vi "LED card.vi"(8 "error in (no error)":errorcluster, 11 "Node Ptr":T5 format="%.0x") -> (0 "error out":errorcluster)   [LabVIEW 2014, in "SLSC configuration System Explorer.lvlib"]
uses:
  SLSC configuration System Explorer.lvlib
  <vilib>/NI Veristand/Custom Device API/Custom Device Item Ref.ctl
  Type Defs/Card Position.ctl
  Shared/SPI Utility/Slot #.ctl
  Shared/LED Backplane/Bank LED States.ctl
  Shared/LED Backplane/LED State.ctl
  Shared/Constants.vi
  <vilib>/NI Veristand/Custom Device API/Get Item Property (U16).vi
  <vilib>/NI Veristand/Custom Device API/Custom Device API.lvlib
  Shared/SLSC configuration Shared.lvlib
panel:
  in  "Bank LED States":T1
  in  "Header 2":cluster{"Section Name":string}={"Section Name"="Bank 0 Settings"}
  in  "Card Position":T3 {"Slot #" max=15}
  in  "Header":cluster{"Section Name":string}={"Section Name"="LED Backplane Settings"}
  in  "Description":string
  in  "Name":string
  # "LED 1"
  # "LED 2"
  # "LED 3"
  # "LED 4"
  # "LED 5"
  # "LED 6"
  # "LED 7"
  # "LED 8"
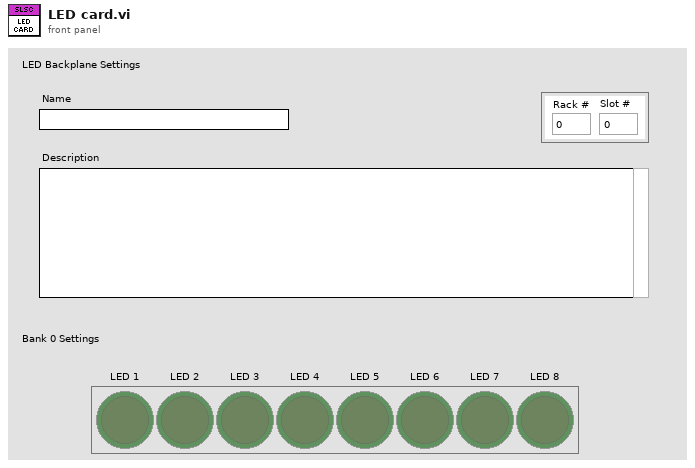
[diagram p1: front panel]
types:
  T1 = typedef "SLSC configuration Shared.lvlib/Bank LED States.ctl" = T2[]
  T2 = typedef "SLSC configuration Shared.lvlib/LED State.ctl" = bool
  T3 = typedef "SLSC configuration Shared.lvlib/Card Position.ctl" = cluster{"Rack #":u8, "Slot #":T4}
  T4 = typedef "SLSC configuration Shared.lvlib/Slot #.ctl" = u8
  T5 = typedef "Custom Device API.lvlib/Custom Device Item Ref.ctl" = u64
  T6 = typedef "Custom Device API.lvlib/Custom Device Commands.ctl" = enum16{"Default", "Item renamed", "Shutdown", "Dynamic button pressed"}
  T7 = typedef "Custom Device API.lvlib/Custom Device Item Info.ctl" = cluster{"Name":string, "Is Channel":bool, "GUID":string, "Is Waveform":bool}
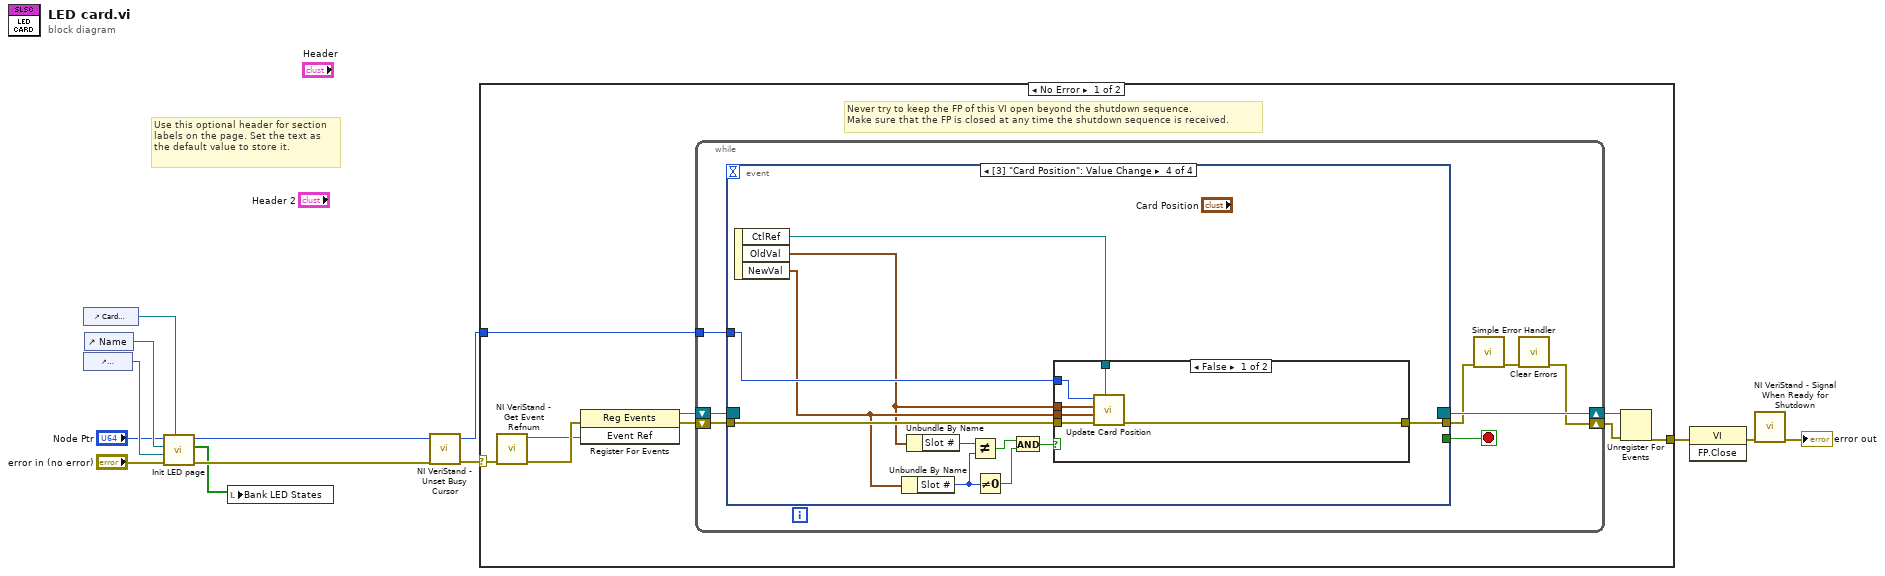
[diagram p0: block diagram]
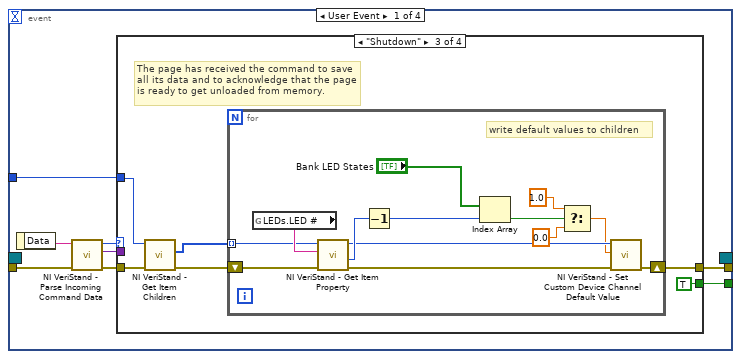
[diagram p2: hidden frame]
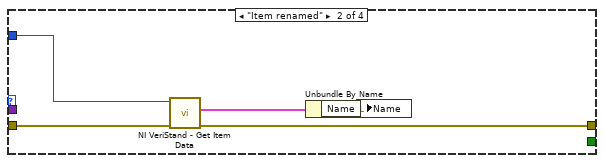
[diagram p4: hidden frame]
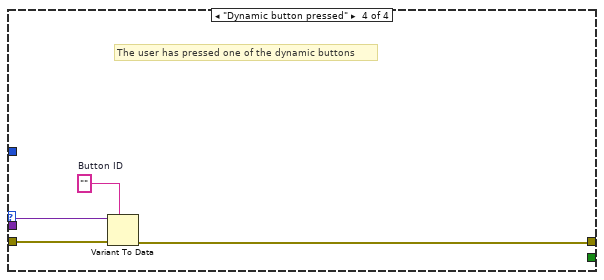
[diagram p5: hidden frame]
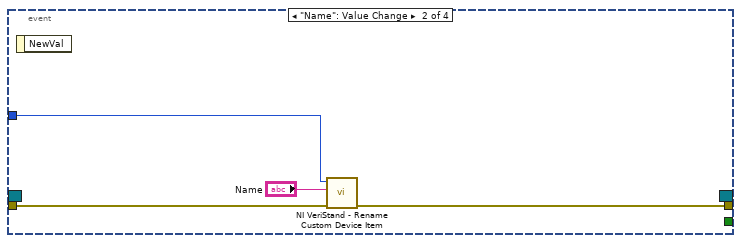
[diagram p6: hidden frame]
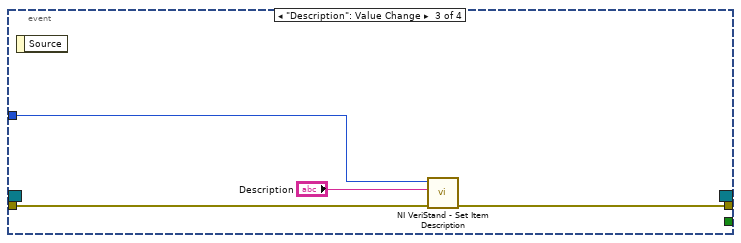
[diagram p7: hidden frame]
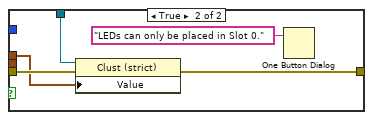
[diagram p8: hidden frame]
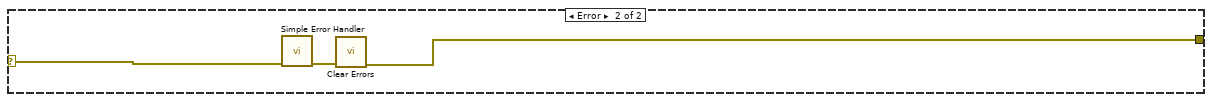
[diagram p9: hidden frame]
diagram:
  # "Use this optional header for section labels on the page. Set the text as the default value to store it."
  n1 = control-ref of="Card Position"() -> (w2:refnum<vi>)
  n2 = control-ref of="Description"() -> (w4:refnum<vi>)
  n3 = control-ref of="Name"() -> (w5:refnum<vi>)
  n4 = call "Init LED page.vi"("Card Position"=w2, "error in (no error)"="error in (no error)", "Description"=w4, "Name"=w5, "Node Ptr"="Node Ptr") -> ("error out"=w9:errorcluster, "LED States"=w1:T2[], "Node Ptr out"=w6:T5)  [unwired: 4 in]
  n5 = local write "Bank LED States"(w1) -> ()
  n6 = call <vilib>:"NI VeriStand - Unset Busy Cursor.vi"("error in (no error)"=w9) -> ("error out"=w8:errorcluster)  [unwired: 10 out]
  n7 = case shown="No Error" w8 {
    selector: w8 -> [w13 w99]
    tunnel: [w18 w97] -> w12
    tunnel: w6 -> [w14 _]
    frame No Error {
      # "Never try to keep the FP of this VI open beyond the shutdown sequence.\nMake sure that the FP is closed at any time the shutdown sequence is received."
      n8 = call <vilib>:"NI VeriStand - Get Event Refnum.vi"("error in (no error)"=w13) -> ("error out"=w21:errorcluster, "Event Ref"=w17:refnum<user-event>)  [unwired: 9 out]
      n9 = register-events(error in=w21, w17) -> (reference out=w15:refnum<event-registration>, error out=w16:errorcluster)  [unwired: 1 in]
      n10 = while {
        tunnel: w14 -> [w25]
        shift-right: [w22] -> w19
        shift-left: w16 -> [w28]
        shift-right: [w29] -> w20
        shift-left: w15 -> [w27]
        stop <- w26 stop-if-true
        n11 = event shown="[3] \"Card Position\": Value Change" {
          selector: w27 -> [_ _ _ _]
          dyn-events: [_ _ _ _] -> w29
          timeout: _ -> [_ _ _ _]
          tunnel: w28 -> [w37 w70 w73 w84]
          tunnel: [w33 _ _ _] -> w26
          tunnel: [w32 w69 w72 w85] -> w24
          tunnel: w25 -> [w31 w68 w74 w83]
          event User Event {
            n12 = event-data() -> ("Data"=w36:string)  [unwired: 1 out]
            n13 = call <vilib>:"NI VeriStand - Parse Incoming Command Data.vi"("error in (no error)"=w37, "Incoming data"=w36) -> ("error out"=w35:errorcluster, "Outgoing data"=w30:variant, "Action"=w34:T6)  [unwired: 7 out]
            n14 = case shown="\"Shutdown\"" w34 {
              tunnel: w35 -> [w38 w43 w46 w66]
              tunnel: [_ _ TRUE _] -> w33
              tunnel: [w38 w40 w48 w63] -> w32
              tunnel: w31 -> [_ w42 w44 _]
              tunnel: w30 -> [_ _ _ w65]
              frame "Default", Default {
              }
              frame "Item renamed" {
                n15 = call <vilib>:"NI VeriStand - Get Item Data.vi"("error in (no error)"=w43, "Item Ref in"=w42) -> ("error out"=w40:errorcluster, "Item Info"=w41:T7)  [unwired: 8 out]
                n16 = Unbundle By Name(w41) -> ("Name"=w39:string)
                n17 = local write "Name"(w39) -> ()
              }
              frame "Shutdown" {
                # "The page has received the command to save all its data and to acknowledge that the page is ready to get unloaded from memory."
                n18 = call <vilib>:"NI VeriStand - Get Item Children.vi"("error in (no error)"=w46, "Item Ref in"=w44) -> ("error out"=w45:errorcluster, "Child Refs"=w47:T5[])  [unwired: 6 in, 2 out]
                n19 = for {
                  shift-right: [w59] -> w48
                  shift-left: w45 -> [w61]
                  tunnel: w47 -> [w57] mode=indexing
                  # "write default values to children"
                  n20 = global read "Constants.vi" "LEDs.LED #"() -> (w62:string)
                  n21 = call-poly <vilib>:"NI VeriStand - Get Item Property.vi"("error in (no error)"=w61, "Property Name"=w62, "Item Ref in"=w57) -> ("error out"=w55:errorcluster, "Value"=w60:u16, "Item Ref out"=w58:T5)  [unwired: 5 in, 1 out]
                  n22 = Decrement(x=w60) -> (x-1=w56:u16)
                  n23 = Index Array(array="Bank LED States", index=w56) -> (element=w53:T2)
                  n24 = Select(t=1.0 ("double precision float"), s=w53, f=0.0 ("double precision float")) -> (s? t:f=w50:dbl)
                  n25 = call <vilib>:"NI VeriStand - Set Custom Device Channel Default Value.vi"("error in (no error)"=w55, "Default Value"=w50, "Channel Ref in"=w58) -> ("error out"=w59:errorcluster)  [unwired: 7 in, 1 out]
                }
              }
              frame "Dynamic button pressed" {
                w64 = ""  # Button ID
                # "The user has pressed one of the dynamic buttons"
                n26 = Variant To Data(error in=w66, type=w64, Variant=w65) -> (error out=w63:errorcluster)  [unwired: 1 out]
              }
            }
          }
          event "Name": Value Change {
            n27 = event-data() -> ()  [unwired: 2 out]
            n28 = call <vilib>:"NI VeriStand - Rename Custom Device Item.vi"("error in (no error)"=w70, "New Name"="Name", "Item Ref in"=w68) -> ("error out"=w69:errorcluster)  [unwired: 1 in, 7 out]
          }
          event "Description": Value Change {
            n29 = event-data() -> ()  [unwired: 2 out]
            n30 = call <vilib>:"NI VeriStand - Set Item Description.vi"("error in (no error)"=w73, "Description"="Description", "Item Ref in"=w74) -> ("error out"=w72:errorcluster)  [unwired: 8 out]
          }
          event Value Change {
            n31 = event-data() -> ("CtlRef"=w82:refnum<vi>, "OldVal"=w80:T3, "NewVal"=w81:T3)  [unwired: 1 out]
            n32 = Unbundle By Name(w81) -> ("Slot #"=w78:T4)
            n33 = Unbundle By Name(w80) -> ("Slot #"=w79:T4)
            n34 = Not Equal?(x=w79, y=w78) -> (x != y?=w75:bool)
            n35 = Not Equal To 0?(x=w78) -> (x != 0?=w77:bool)
            n36 = And(x=w75, y=w77) -> (x .and. y?=w76:bool)
            n37 = case shown="False" w76 {
              tunnel: [w91 w96] -> w85
              tunnel: w84 -> [w90 w95]
              tunnel: w80 -> [w89 w93]
              tunnel: w83 -> [w88 _]
              tunnel: w82 -> [w87 w94]
              tunnel: w81 -> [w86 _]
              frame False {
                n38 = call "Update Card Position.vi"("Card Position Ref"=w87, "error in (no error)"=w90, "NewVal"=w86, "OldVal"=w89, "Node Ptr in"=w88) -> ("error out"=w91:errorcluster)  [unwired: 6 in]
              }
              frame True {
                n39 = property class="Clust (strict)"(reference=w94, error in=w95, "Value"=w93) -> (error out=w96:errorcluster)  [unwired: 1 out]
                n40 = One Button Dialog(message="LEDs can only be placed in Slot 0.") -> ()  [unwired: 1 in, 1 out]
              }
            }
          }
        }
        n41 = call <vilib>:"Simple Error Handler.vi"("error in (no error)"=w24) -> ("error out"=w23:errorcluster)  [unwired: 1 in, 7 out]
        n42 = call <vilib>:"Clear Errors.vi"("error in (no error)"=w23) -> ("error out"=w22:errorcluster)  [unwired: 1 in, 5 out]
      }
      n43 = Unregister For Events(event registration refnum=w20, error in=w19) -> (error out=w18:errorcluster)
    }
    frame Error {
      n44 = call <vilib>:"Simple Error Handler.vi"("error in (no error)"=w99) -> ("error out"=w98:errorcluster)  [unwired: 1 in, 7 out]
      n45 = call <vilib>:"Clear Errors.vi"("error in (no error)"=w98) -> ("error out"=w97:errorcluster)  [unwired: 1 in, 5 out]
    }
  }
  n46 = invoke class="VI" method="FP.Close"(error in=w12) -> (error out=w11:errorcluster)  [unwired: 2 in, 2 out]
  n47 = call <vilib>:"NI VeriStand - Signal When Ready for Shutdown.vi"("error in (no error)"=w11) -> ("error out"=→"error out":errorcluster)  [unwired: 10 out]
